vi "Mover4_Model_DHdefinition_modified.vi"(8 "error in":errorcluster) -> (0 "error out":errorcluster, 3 "serial arm out":refnum<class "NI_Robotics_6R Type 1 Serial Arm Class.lvclass">)   [LabVIEW 2015]
uses:
  <vilib>/robotics/Kinematics/Analytical/6R/Type 1/NI_Robotics_6R Type 1 Serial Arm Class.lvclass
  <vilib>/robotics/Kinematics/Link/Joint Type.ctl
  <vilib>/Analysis/coordinate.llb/Euler Angles To Direction Cosines.vi
  <vilib>/robotics/Kinematics/Analytical/6R/Type 1/Initialize 6R Type 1 Serial Arm.vi
  <vilib>/robotics/Kinematics/Robot/NI_Robotics_Serial Robot Arm.lvclass
  <vilib>/robotics/Kinematics/NI_Kinematics.lvlib
  <vilib>/robotics/Kinematics/Analytical/NI_Robotics_AnalyticKinematics.lvlib
  <vilib>/robotics/Kinematics/Link/NI_Robotics_Link.lvclass
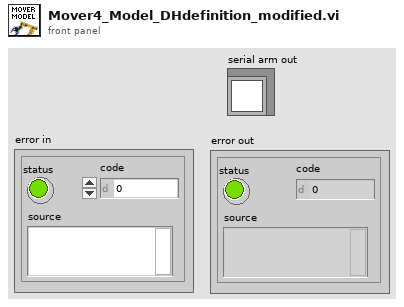
[diagram p1: front panel]
types:
  T1 = typedef "NI_Robotics_Link.lvclass/Joint Type.ctl" = enum16{"Revolute", "Prismatic"}
  T2 = cluster{"Twist Angle":dbl, "Length":dbl, "Rotation Angle":dbl, "Offset Distance":dbl, "Joint Type":T1, "Joint Coordinate Offset":dbl}[]
  T3 = typedef "NI_Matrix.lvlib/RealMatrix.ctl" = dbl[][]
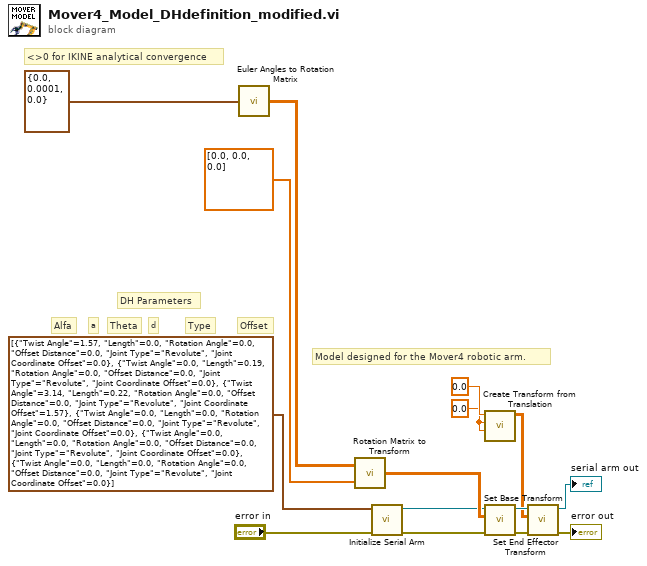
[diagram p0: block diagram]
diagram:
  w4 = 0.0 ("z")
  # "Offset"
  # "Type"
  # "Model designed for the Mover4 robotic arm."
  # "<>0 for IKINE analytical convergence"
  # "d"
  # "Theta"
  # "a"
  # "Alfa"
  # "DH Parameters"
  n1 = call <vilib>:"Euler Angles to Rotation Matrix.vi"("euler angles"=cluster{"roll":dbl, "pitch":dbl, "yaw":dbl} {"roll"=0.0, "pitch"=0.0001, "yaw"=0.0} ("angles")) -> ("rotation matrix"=w14:T3)
  n2 = call <vilib>:"Rotation Matrix to Transform.vi"("translation vector"=dbl[] [0.0, 0.0, 0.0], "rotation matrix"=w14) -> ("transform"=w12:T3)
  n3 = call-poly <vilib>:"Initialize Serial Arm.vi"("error in (no error)"="error in", "kinematic parameters"=T2 [{"Twist Angle"=1.57, "Length"=0.0, "Rotation Angle"=0.0, "Offset Distance"=0.0, "Joint Type"=enum."Revolute", "Joint Coordinate Offset"=0.0}, {"Twist Angle"=0.0, "Length"=0.19, "Rotation Angle"=0.0, "Offset Distance"=0.0, "Joint Type"=enum."Revolute", "Joint Coordinate Offset"=0.0}, {"Twist Angle"=3.14, "Length"=0.22, "Rotation Angle"=0.0, "Offset Distance"=0.0, "Joint Type"=enum."Revolute", "Joint Coordinate Offset"=1.57}, {"Twist Angle"=0.0, "Length"=0.0, "Rotation Angle"=0.0, "Offset Distance"=0.0, "Joint Type"=enum."Revolute", "Joint Coordinate Offset"=0.0}, {"Twist Angle"=0.0, "Length"=0.0, "Rotation Angle"=0.0, "Offset Distance"=0.0, "Joint Type"=enum."Revolute", "Joint Coordinate Offset"=0.0}, {"Twist Angle"=0.0, "Length"=0.0, "Rotation Angle"=0.0, "Offset Distance"=0.0, "Joint Type"=enum."Revolute", "Joint Coordinate Offset"=0.0}] ("kinematics parameters")) -> ("error out"=w11:errorcluster, "6R type 1 serial arm out"=w10:refnum<class "NI_Robotics_6R Type 1 Serial Arm Class.lvclass">)  [unwired: 8 in]
  n4 = call <vilib>:"Create Transform from Translation.vi"("z"=w4, "y"=w4, "x"=0.0) -> ("transform"=w3:T3)  [unwired: 8 in]
  n5 = call <vilib>:"Set Base Transform.vi"("error in (no error)"=w11, "base transform"=w12, "serial arm in"=w10) -> ("error out"=w8:errorcluster, "serial arm out"=w9:refnum<class "NI_Robotics_6R Type 1 Serial Arm Class.lvclass">)  [unwired: 7 in]
  n6 = call <vilib>:"Set End Effector Transform.vi"("error in (no error)"=w8, "end effector transform"=w3, "serial arm in"=w9) -> ("error out"=→"error out":errorcluster, "serial arm out"=→"serial arm out":refnum<class "NI_Robotics_6R Type 1 Serial Arm Class.lvclass">)  [unwired: 7 in]
